vi "PathPlanner_PathFinder_UpdateState.vi"(6 "Closed":set{T1}(c389), 7 "S":T1, 8 "G":map{i32, dbl}(c390), 9 "Incons":map{i32, T2}(c390), 10 "Open":map{i32, T2}(c390), 11 "RHS":map{i32, dbl}(c390)) -> (1 "Incons out":map{i32, T2}(c390), 2 "Open out":map{i32, T2}(c390), 3 "RHS out":map{i32, dbl}(c390))   [LabVIEW 2019, in "PathPlanner24.lvlib"]
uses:
  TypeDef/PathPlannerFinderGridPosition.ctl
  PathPlanner_GridPosition_Get.vi
  PathPlanner_PathFinder_Globals.vi
  PathPlanner24.lvlib
  TypeDef/PathPlannerFinderDoublePair.ctl
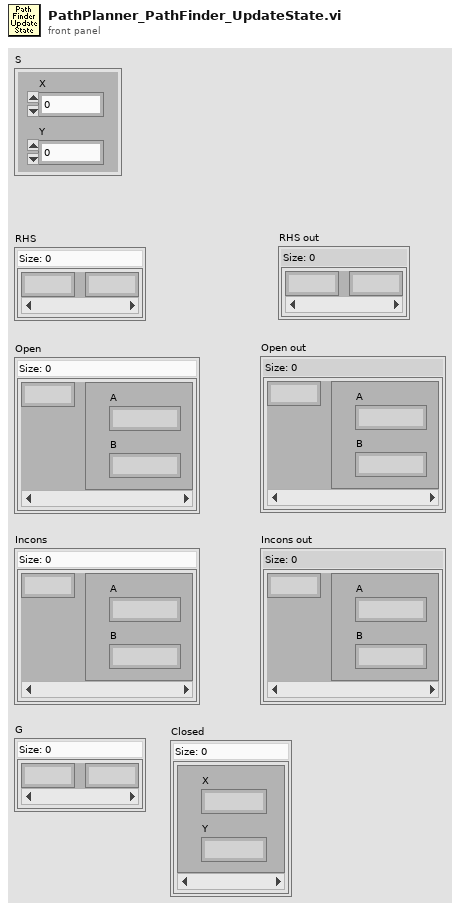
[diagram p1: front panel]
types:
  T1 = typedef "PathPlanner24.lvlib/PathPlannerFinderGridPosition.ctl" = cluster{"X":i32, "Y":i32}
  T2 = typedef "PathPlanner24.lvlib/PathPlannerFinderDoublePair.ctl" = cluster{"A":dbl, "B":dbl}
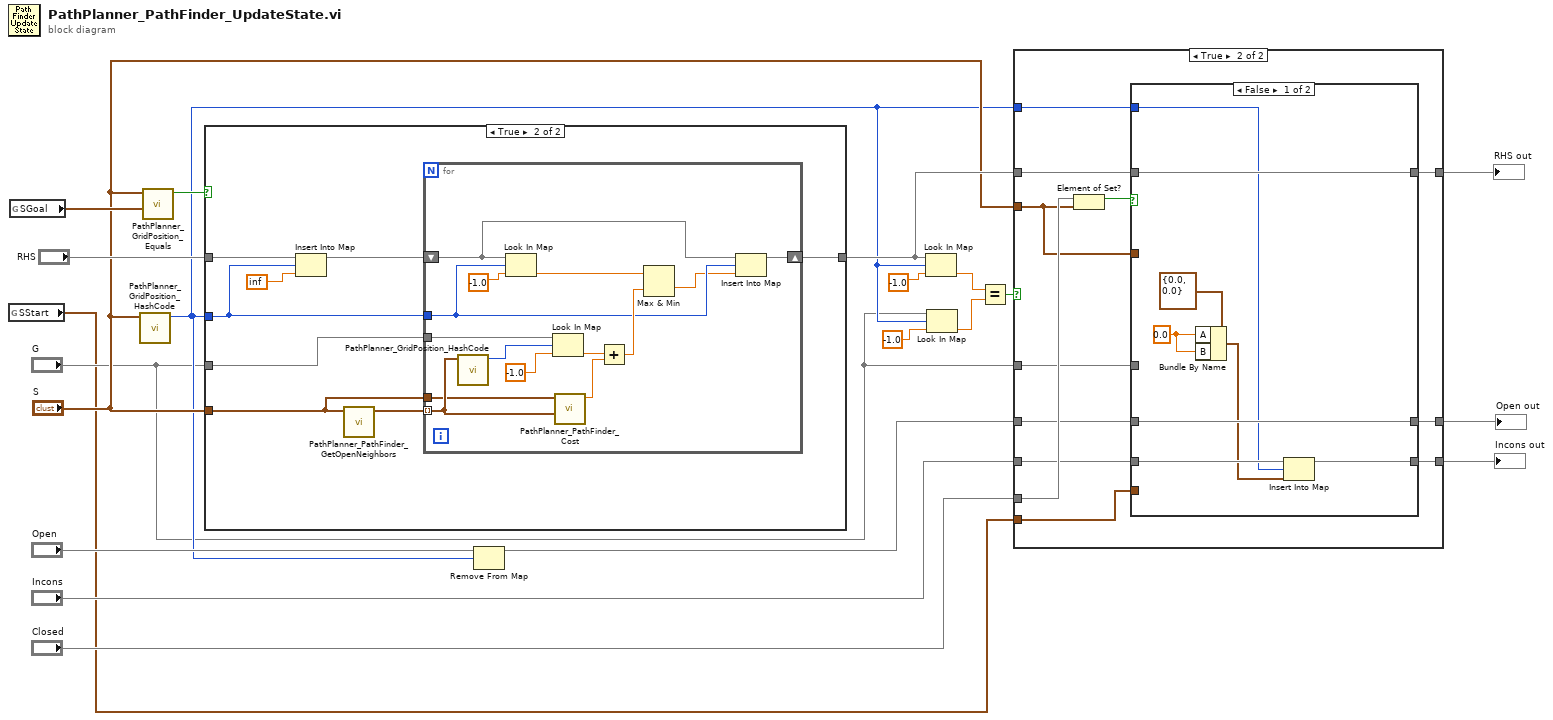
[diagram p0: block diagram]
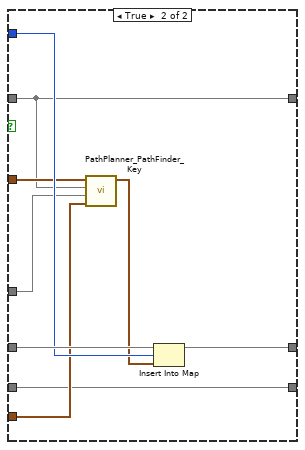
[diagram p3: hidden frame]
diagram:
  n1 = global read "PathPlanner_PathFinder_Globals.vi" "SStart"() -> (w1:T1)
  n2 = global read "PathPlanner_PathFinder_Globals.vi" "SGoal"() -> (w20:T1)
  n3 = call "PathPlanner_GridPosition_HashCode.vi"("GridPosition"="S") -> ("HashCode"=w3:i32)  [unwired: 10 in]
  n4 = call "PathPlanner_GridPosition_Equals.vi"("Other GridPosition"=w20, "GridPosition"="S") -> ("Equal"=w19:bool)  [unwired: 9 in]
  n5 = case shown="True" w19 {
    tunnel: "RHS" -> [w21 w29]
    tunnel: w3 -> [_ w25]
    tunnel: "S" -> [_ w23]
    tunnel: "G" -> [_ w24]
    tunnel: [w21 w22] -> w9
    frame False {
    }
    frame True {
      n6 = Insert Into Map(map in=w29, key=w25, value=inf) -> (map out=w26:map{i32, dbl})  [unwired: 2 out]
      n7 = call "PathPlanner_PathFinder_GetOpenNeighbors.vi"("GridPosition S"=w23) -> ("Neighbors"=w27:T1[])  [unwired: 10 in]
      n8 = for {
        tunnel: w27 -> [w36] mode=indexing
        shift-right: [w30] -> w22
        shift-left: w26 -> [w33]
        tunnel: w25 -> [w32]
        tunnel: w24 -> [w42]
        tunnel: w23 -> [w35]
        n9 = call "PathPlanner_GridPosition_HashCode.vi"("GridPosition"=w36) -> ("HashCode"=w41:i32)  [unwired: 10 in]
        n10 = Look In Map(map=w33, key=w32, default value=-1.0) -> (value=w39:dbl)  [unwired: 1 out]
        n11 = Look In Map(map=w42, key=w41, default value=-1.0) -> (value=w37:dbl)  [unwired: 1 out]
        n12 = call "PathPlanner_PathFinder_Cost.vi"("sGoal"=w36, "sStart"=w35) -> ("Cost"=w38:dbl)  [unwired: 9 in]
        n13 = Add(x=w37, y=w38) -> (x+y=w34:dbl)
        n14 = Max & Min(x=w39, y=w34) -> (min(x,y)=w31:dbl)  [unwired: 1 out]
        n15 = Insert Into Map(map in=w33, key=w32, value=w31) -> (map out=w30:map{i32, dbl})  [unwired: 2 out]
      }
    }
  }
  n16 = Remove From Map(10:w3, 11:"Open") -> (3:w12:map{i32, T2})  [unwired: 2 out]
  n17 = Look In Map(map=w9, key=w3, default value=-1.0) -> (value=w14:dbl)  [unwired: 1 out]
  n18 = Look In Map(map="G", key=w3, default value=-1.0) -> (value=w13:dbl)  [unwired: 1 out]
  n19 = Equal?(x=w14, y=w13) -> (x = y?=w10:bool)
  n20 = case shown="True" w10 {
    tunnel: w12 -> [w45 w56]
    tunnel: "Incons" -> [w44 w48]
    tunnel: w9 -> [w46 w53]
    tunnel: [w46 w49] -> w8
    tunnel: [w45 w50] -> w7
    tunnel: [w44 w47] -> w6
    tunnel: "Closed" -> [_ w58]
    tunnel: "S" -> [_ w54]
    tunnel: w3 -> [_ w55]
    tunnel: "G" -> [_ w52]
    tunnel: w1 -> [_ w51]
    frame False {
    }
    frame True {
      n21 = Element of Set?(10:w54, 11:w58) -> (3:w57:bool)
      n22 = case shown="False" w57 {
        tunnel: w56 -> [w63 w75]
        tunnel: w55 -> [w62 w74]
        tunnel: w54 -> [_ w73]
        tunnel: w53 -> [w64 w68]
        tunnel: w52 -> [_ w72]
        tunnel: w51 -> [_ w71]
        tunnel: [w63 w69] -> w50
        tunnel: [w64 w68] -> w49
        tunnel: w48 -> [w66 w67]
        tunnel: [w65 w67] -> w47
        frame False {
          w60 = 0.0 ("A")
          n23 = Bundle By Name(cluster=T2 {"A"=0.0, "B"=0.0} ("PathPlannerFinderDoublePair"), "A"=w60, "B"=w60) -> (w59:T2)
          n24 = Insert Into Map(map in=w66, key=w62, value=w59) -> (map out=w65:map{i32, T2})  [unwired: 2 out]
        }
        frame True {
          n25 = call "PathPlanner_PathFinder_Key.vi"("Sstart"=w71, "G"=w72, "RHS"=w68, "S"=w73) -> ("DoublePair"=w70:T2)  [unwired: 7 in]
          n26 = Insert Into Map(map in=w75, key=w74, value=w70) -> (map out=w69:map{i32, T2})  [unwired: 2 out]
        }
      }
    }
  }
  "RHS out" <- w8
  "Open out" <- w7
  "Incons out" <- w6
